vi "Text2Cluster.vi"(11 "string":string) -> (1 "# of Errors":i32, 2 "remainder":string, 3 "Log":T3={"Sent"="", "Reply"="", "Method Name"="", "success"=FALSE, "Dir1"="", "Dir2"="", "Error Information"="", "VI Name"="", "ROS"={"topic port"=0, "Node"="", "topic"="", "type"="", "node port"=0, "error "={"status"=FALSE, "code"=0, "source"=""}, "Direction"=enum."Node", "APIs"=[], "Update (ms)"=1, "write queue"=1}, "close reference"={"status"=FALSE, "code"=0, "source"=""}, "release queue"={"status"=FALSE, "code"=0, "source"=""}, "release notification"={"status"=FALSE, "code"=0, "source"=""}, "varaiant to data"={"status"=FALSE, "code"=0, "source"=""}, "console error"={"status"=FALSE, "code"=0, "source"=""}, "Time Stamp"=""})   [LabVIEW 2012]
uses:
  <userlib>/ROSforLV/ROS/Code/SubVIs/_ROSControl.ctl
  <userlib>/ROSforLV/ROS/Code/SubVIs/_ROSDirection.ctl
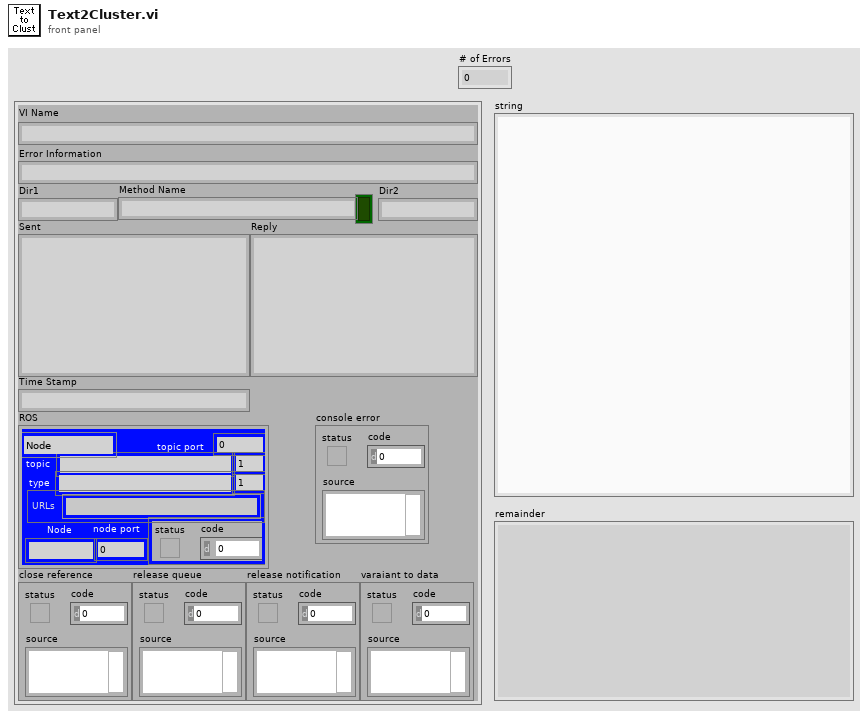
[diagram p1: front panel]
types:
  T1 = typedef "_ROSControl.ctl" = cluster{"topic port":u16, "Node":string, "topic":string, "type":string, "node port":u32, "error ":errorcluster, "Direction":T2, "APIs":string[], "Update (ms)":u16, "write queue":u16}
  T2 = typedef "_ROSDirection.ctl" = enum16{"Node", "Publisher", "Subscriber", "Service Client"}
  T3 = cluster{"Sent":string, "Reply":string, "Method Name":string, "success":bool, "Dir1":string, "Dir2":string, "Error Information":string, "VI Name":string, "ROS":T1, "close reference":errorcluster, "release queue":errorcluster, "release notification":errorcluster, "varaiant to data":errorcluster, "console error":errorcluster, "Time Stamp":string}
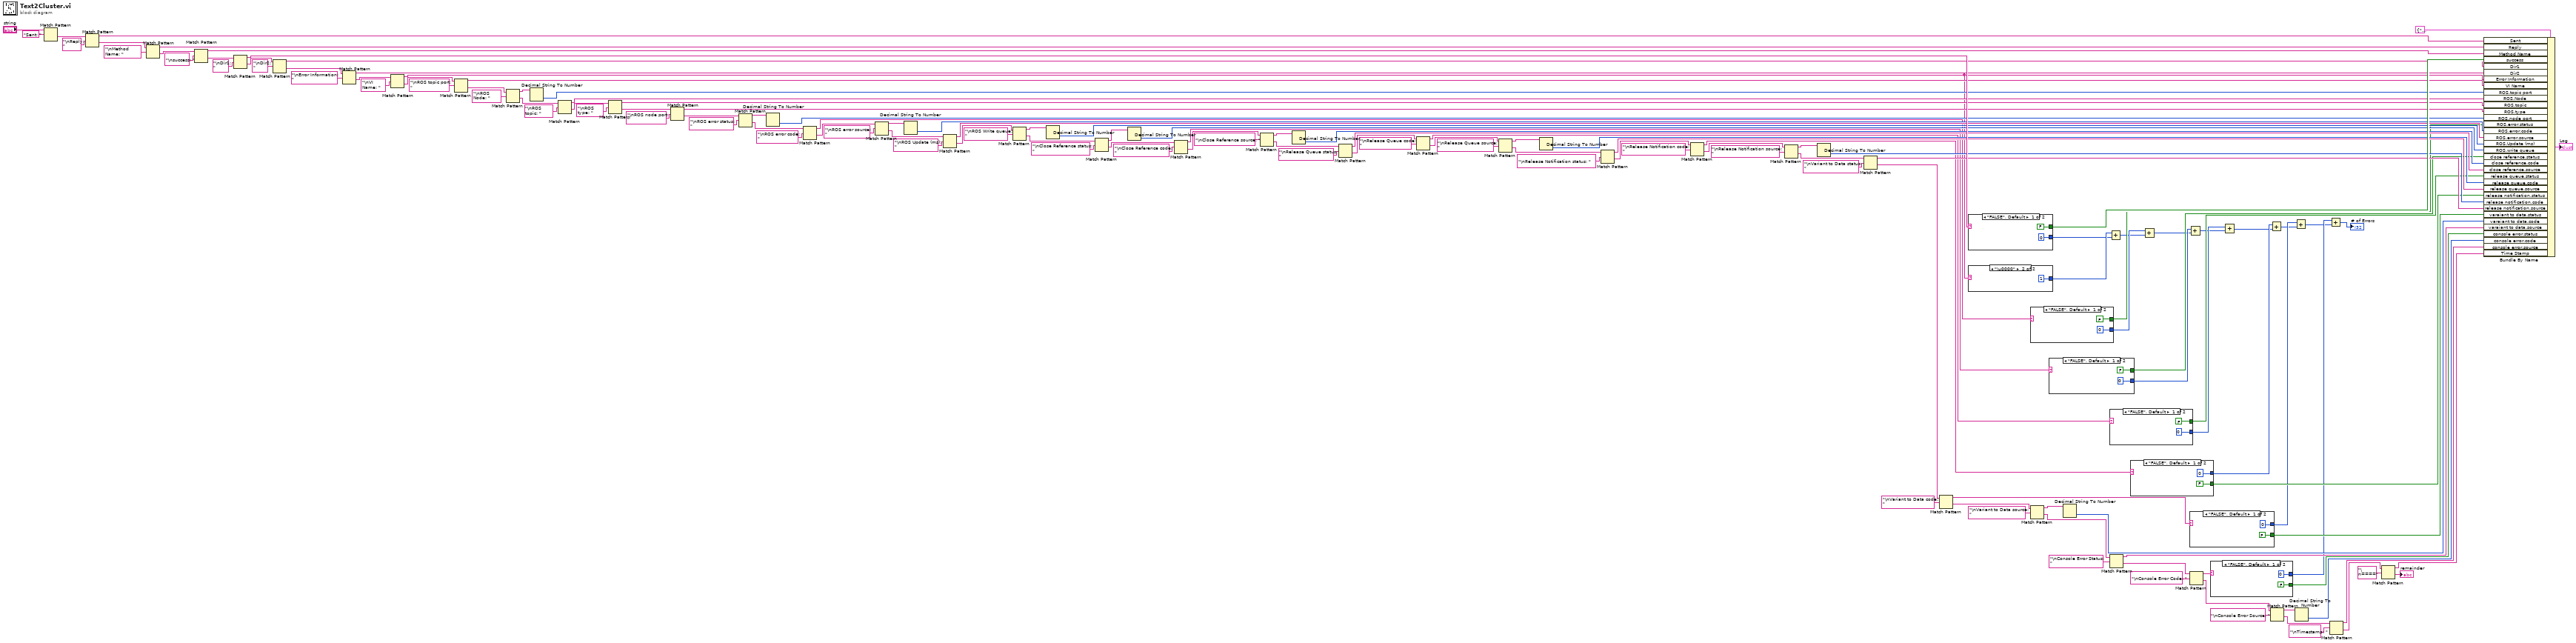
[diagram p0: block diagram]
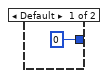
[diagram p2: hidden frame]
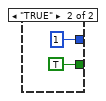
[diagram p3: hidden frame]
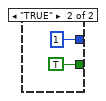
[diagram p4: hidden frame]
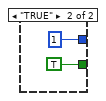
[diagram p5: hidden frame]
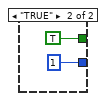
[diagram p6: hidden frame]
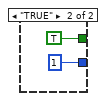
[diagram p7: hidden frame]
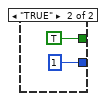
[diagram p8: hidden frame]
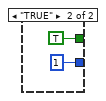
[diagram p9: hidden frame]
diagram:
  n1 = Match Pattern(string="string", regular expression="Sent: ") -> (after substring=w136:string)  [unwired: 1 in, 3 out]
  n2 = Match Pattern(string=w136, regular expression="\nReply: ") -> (before substring=w70:string, after substring=w127:string)  [unwired: 1 in, 2 out]
  n3 = Match Pattern(string=w127, regular expression="\nMethod Name: ") -> (before substring=w69:string, after substring=w126:string)  [unwired: 1 in, 2 out]
  n4 = Match Pattern(string=w126, regular expression="\nsuccess: ") -> (before substring=w68:string, after substring=w125:string)  [unwired: 1 in, 2 out]
  n5 = Match Pattern(string=w125, regular expression="\nDir1: ") -> (before substring=w66:string, after substring=w124:string)  [unwired: 1 in, 2 out]
  n6 = Match Pattern(string=w124, regular expression="\nDir2: ") -> (before substring=w65:string, after substring=w123:string)  [unwired: 1 in, 2 out]
  n7 = Match Pattern(string=w123, regular expression="\nError Information: ") -> (before substring=w64:string, after substring=w122:string)  [unwired: 1 in, 2 out]
  n8 = Match Pattern(string=w122, regular expression="\nVI Name: ") -> (before substring=w4:string, after substring=w121:string)  [unwired: 1 in, 2 out]
  n9 = Match Pattern(string=w121, regular expression="\nROS topic port: ") -> (before substring=w63:string, after substring=w120:string)  [unwired: 1 in, 2 out]
  n10 = Match Pattern(string=w120, regular expression="\nROS Node: ") -> (before substring=w62:string, after substring=w112:string)  [unwired: 1 in, 2 out]
  n11 = Decimal String To Number(string=w62) -> (number=w61:i32)  [unwired: 2 in, 1 out]
  n12 = Match Pattern(string=w112, regular expression="\nROS topic: ") -> (before substring=w60:string, after substring=w111:string)  [unwired: 1 in, 2 out]
  n13 = Match Pattern(string=w111, regular expression="\nROS type: ") -> (before substring=w59:string, after substring=w110:string)  [unwired: 1 in, 2 out]
  n14 = Match Pattern(string=w110, regular expression="\nROS node port: ") -> (before substring=w58:string, after substring=w109:string)  [unwired: 1 in, 2 out]
  n15 = Match Pattern(string=w109, regular expression="\nROS error status: ") -> (before substring=w56:string, after substring=w108:string)  [unwired: 1 in, 2 out]
  n16 = Decimal String To Number(string=w56) -> (number=w57:i32)  [unwired: 2 in, 1 out]
  n17 = Match Pattern(string=w108, regular expression="\nROS error code: ") -> (before substring=w28:string, after substring=w107:string)  [unwired: 1 in, 2 out]
  n18 = Match Pattern(string=w107, regular expression="\nROS error source: ") -> (before substring=w54:string, after substring=w106:string)  [unwired: 1 in, 2 out]
  n19 = Decimal String To Number(string=w54) -> (number=w55:i32)  [unwired: 2 in, 1 out]
  n20 = Match Pattern(string=w106, regular expression="\nROS Update (ms): ") -> (before substring=w53:string, after substring=w72:string)  [unwired: 1 in, 2 out]
  n21 = Match Pattern(string=w72, regular expression="\nROS Write queue: ") -> (before substring=w52:string, after substring=w98:string)  [unwired: 1 in, 2 out]
  n22 = Decimal String To Number(string=w52) -> (number=w50:i32)  [unwired: 2 in, 1 out]
  n23 = Match Pattern(string=w98, regular expression="\nClose Reference status: ") -> (before substring=w51:string, after substring=w97:string)  [unwired: 1 in, 2 out]
  n24 = Decimal String To Number(string=w51) -> (number=w49:i32)  [unwired: 2 in, 1 out]
  n25 = Match Pattern(string=w97, regular expression="\nClose Reference code: ") -> (before substring=w25:string, after substring=w96:string)  [unwired: 1 in, 2 out]
  n26 = Match Pattern(string=w96, regular expression="\nClose Reference source: ") -> (before substring=w47:string, after substring=w95:string)  [unwired: 1 in, 2 out]
  n27 = Decimal String To Number(string=w47) -> (number=w48:i32)  [unwired: 2 in, 1 out]
  n28 = Match Pattern(string=w95, regular expression="\nRelease Queue status: ") -> (before substring=w46:string, after substring=w94:string)  [unwired: 1 in, 2 out]
  n29 = Match Pattern(string=w94, regular expression="\nRelease Queue code: ") -> (before substring=w24:string, after substring=w93:string)  [unwired: 1 in, 2 out]
  n30 = Match Pattern(string=w93, regular expression="\nRelease Queue source: ") -> (before substring=w45:string, after substring=w88:string)  [unwired: 1 in, 2 out]
  n31 = Decimal String To Number(string=w45) -> (number=w44:i32)  [unwired: 2 in, 1 out]
  n32 = Match Pattern(string=w88, regular expression="\nRelease Notification status: ") -> (before substring=w43:string, after substring=w90:string)  [unwired: 1 in, 2 out]
  n33 = Match Pattern(string=w90, regular expression="\nRelease Notification code: ") -> (before substring=w22:string, after substring=w89:string)  [unwired: 1 in, 2 out]
  n34 = Match Pattern(string=w89, regular expression="\nRelease Notification source: ") -> (before substring=w42:string, after substring=w83:string)  [unwired: 1 in, 2 out]
  n35 = Decimal String To Number(string=w42) -> (number=w41:i32)  [unwired: 2 in, 1 out]
  n36 = Match Pattern(string=w83, regular expression="\nVariant to Data status: ") -> (before substring=w40:string, after substring=w85:string)  [unwired: 1 in, 2 out]
  n37 = Match Pattern(string=w85, regular expression="\nVariant to Data code: ") -> (before substring=w20:string, after substring=w84:string)  [unwired: 1 in, 2 out]
  n38 = case shown="\"FALSE\", Default" w66 {
    tunnel: [FALSE TRUE] -> w67
    tunnel: [0 1] -> w2
    frame "FALSE", Default {
    }
    frame "TRUE" {
    }
  }
  n39 = case shown="\"\"" w4 {
    tunnel: [0 1] -> w3
    frame Default {
    }
    frame "\u0000" {
    }
  }
  n40 = case shown="\"FALSE\", Default" w28 {
    tunnel: [FALSE TRUE] -> w27
    tunnel: [0 1] -> w12
    frame "FALSE", Default {
    }
    frame "TRUE" {
    }
  }
  n41 = Match Pattern(string=w84, regular expression="\nVariant to Data source: ") -> (before substring=w39:string, after substring=w77:string)  [unwired: 1 in, 2 out]
  n42 = case shown="\"FALSE\", Default" w25 {
    tunnel: [FALSE TRUE] -> w26
    tunnel: [0 1] -> w16
    frame "FALSE", Default {
    }
    frame "TRUE" {
    }
  }
  n43 = Decimal String To Number(string=w39) -> (number=w38:i32)  [unwired: 2 in, 1 out]
  n44 = Add(x=w3, y=w2) -> (x+y=w1:i32)
  n45 = case shown="\"FALSE\", Default" w24 {
    tunnel: [FALSE TRUE] -> w23
    tunnel: [0 1] -> w14
    frame "FALSE", Default {
    }
    frame "TRUE" {
    }
  }
  n46 = Match Pattern(string=w77, regular expression="\nConsole Error Status: ") -> (before substring=w37:string, after substring=w79:string)  [unwired: 1 in, 2 out]
  n47 = case shown="\"FALSE\", Default" w22 {
    tunnel: [FALSE TRUE] -> w21
    tunnel: [0 1] -> w11
    frame "FALSE", Default {
    }
    frame "TRUE" {
    }
  }
  n48 = Add(x=w12, y=w1) -> (x+y=w15:i32)
  n49 = Add(x=w16, y=w15) -> (x+y=w13:i32)
  n50 = case shown="\"FALSE\", Default" w20 {
    tunnel: [FALSE TRUE] -> w19
    tunnel: [0 1] -> w9
    frame "FALSE", Default {
    }
    frame "TRUE" {
    }
  }
  n51 = Match Pattern(string=w79, regular expression="\nConsole Error Code: ") -> (before substring=w18:string, after substring=w78:string)  [unwired: 1 in, 2 out]
  n52 = case shown="\"FALSE\", Default" w18 {
    tunnel: [FALSE TRUE] -> w17
    tunnel: [0 1] -> w7
    frame "FALSE", Default {
    }
    frame "TRUE" {
    }
  }
  n53 = Add(x=w14, y=w13) -> (x+y=w10:i32)
  n54 = Add(x=w11, y=w10) -> (x+y=w8:i32)
  n55 = Match Pattern(string=w78, regular expression="\nConsole Error Source: ") -> (before substring=w35:string, after substring=w74:string)  [unwired: 1 in, 2 out]
  n56 = Add(x=w9, y=w8) -> (x+y=w6:i32)
  n57 = Decimal String To Number(string=w35) -> (number=w34:i32)  [unwired: 2 in, 1 out]
  n58 = Add(x=w7, y=w6) -> (x+y=→"# of Errors":i32)
  n59 = Match Pattern(string=w74, regular expression="\nTimestamp: ") -> (before substring=w36:string, after substring=w31:string)  [unwired: 1 in, 2 out]
  n60 = Match Pattern(string=w31, regular expression="\n====") -> (before substring=w32:string, after substring=→"remainder":string)  [unwired: 1 in, 2 out]
  n61 = Bundle By Name(cluster=T3 {"Sent"="", "Reply"="", "Method Name"="", "success"=FALSE, "Dir1"="", "Dir2"="", "Error Information"="", "VI Name"="", "ROS"={"topic port"=0, "Node"="", "topic"="", "type"="", "node port"=0, "error "={"status"=FALSE, "code"=0, "source"=""}, "Direction"=enum."Node", "APIs"=[], "Update (ms)"=1, "write queue"=1}, "close reference"={"status"=FALSE, "code"=0, "source"=""}, "release queue"={"status"=FALSE, "code"=0, "source"=""}, "release notification"={"status"=FALSE, "code"=0, "source"=""}, "varaiant to data"={"status"=FALSE, "code"=0, "source"=""}, "console error"={"status"=FALSE, "code"=0, "source"=""}, "Time Stamp"=""} ("Log"), "Sent"=w70, "Reply"=w69, "Method Name"=w68, "success"=w67, "Dir1"=w65, "Dir2"=w64, "Error Information"=w4, "VI Name"=w63, "ROS.topic port"=w61, "ROS.Node"=w60, "ROS.topic"=w59, "ROS.type"=w58, "ROS.node port"=w57, "ROS.error.status"=w27, "ROS.error.code"=w55, "ROS.error.source"=w53, "ROS.Update (ms)"=w50, "ROS.write queue"=w49, "close reference.status"=w26, "close reference.code"=w48, "close reference.source"=w46, "release queue.status"=w23, "release queue.code"=w44, "release queue.source"=w43, "release notification.status"=w21, "release notification.code"=w41, "release notification.source"=w40, "varaiant to data.status"=w19, "varaiant to data.code"=w38, "varaiant to data.source"=w37, "console error.status"=w17, "console error.code"=w34, "console error.source"=w36, "Time Stamp"=w32) -> (→"Log":T3)
